vi "Calc speed given dist quadratic but weird.vi"(0 "Distance from dest":dbl=500.0, 5 "Min dist for movement":dbl=50.0, 9 "min speed":dbl=0.3, 11 "error in (no error)":errorcluster, 12 "max speed":dbl=4.0) -> (14 "Speed":dbl, 15 "error out":errorcluster)   [LabVIEW 2016]
panel:
  in  "Distance at speed 4":dbl=300.0
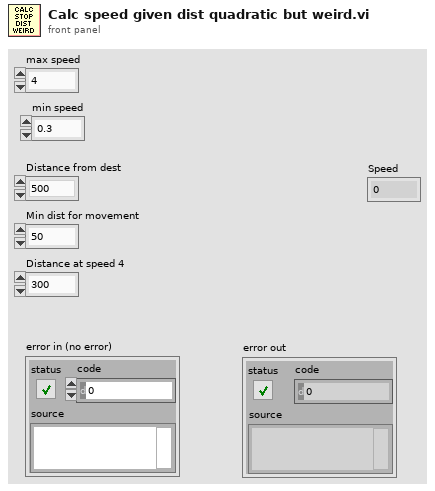
[diagram p1: front panel]
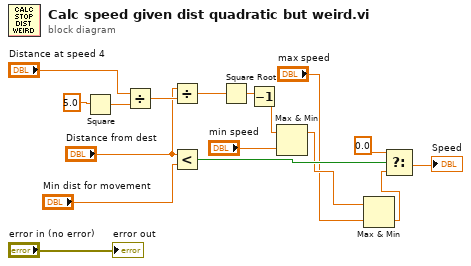
[diagram p0: block diagram]
diagram:
  n1 = Square(x=5.0) -> (x^2=w16:dbl)
  n2 = Divide(x="Distance at speed 4", y=w16) -> (x/y=w13:dbl)
  n3 = Divide(x="Distance from dest", y=w13) -> (x/y=w12:dbl)
  n4 = Less?(x="Distance from dest", y="Min dist for movement") -> (x < y?=w8:bool)
  n5 = Square Root(x=w12) -> (sqrt(x)=w2:dbl)
  n6 = Decrement(x=w2) -> (x-1=w1:dbl)
  n7 = Max & Min(x=w1, y="min speed") -> (max(x,y)=w5:dbl)  [unwired: 1 out]
  n8 = Max & Min(x=w5, y="max speed") -> (min(x,y)=w3:dbl)  [unwired: 1 out]
  n9 = Select(t=0.0, s=w8, f=w3) -> (s? t:f=→"Speed":dbl)
  "error out" <- "error in (no error)"
